vi "FTW-TestExecutive-Core_OnLoadSequence.vi"(0 "FTW-Scripter-Core In":refnum<class "FTW-TestExecutive-Core.lvclass">, 11 "error in":errorcluster) -> (4 "FTW-Scripter-Core Out":refnum<class "FTW-TestExecutive-Core.lvclass">, 15 "error out":errorcluster)   [LabVIEW 2015, in "FTW-TestExecutive-Core.lvclass"]
uses:
  FTW-TestExecutive-Core.lvclass
  FTW-TestExecutive-Core.lvclass/FTW-TestExecutive-Core.ctl
  source/actor/Instance-Extended/FTW-ActorExtended.lvclass
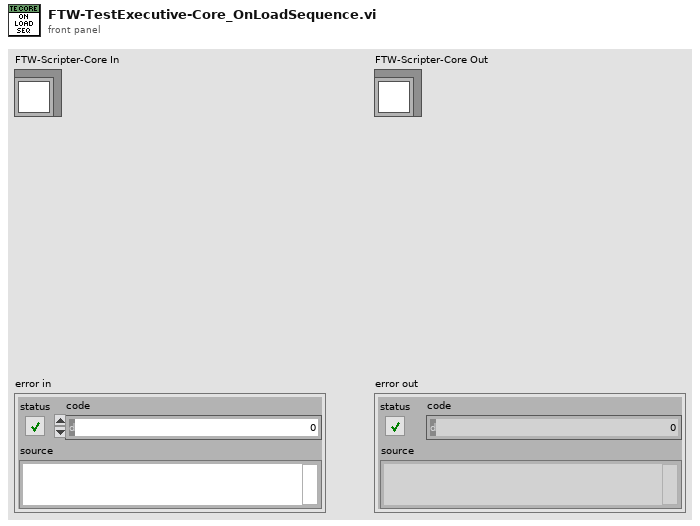
[diagram p1: front panel]
types:
  T1 = typedef "FTW-TestExecutive-Step.ctl" = cluster{"Name":string, "Type":string, "Path":string, "Config":string, "Elapsed Time":dbl, "Passed":bool, "State":T2, "Results":T3}
  T2 = typedef "FTW-TestExecutive-Step-State.ctl" = enum8{"None", "Failed", "Passed", "Timed out", "Aborted"}
  T3 = typedef "FTW-TestExecutive-Results.ctl" = cluster{"Start Time":timestamp, "Elapsed Time":dbl, "Passed":bool, "Additional Results":refnum<class "FTW-Container.lvclass">}
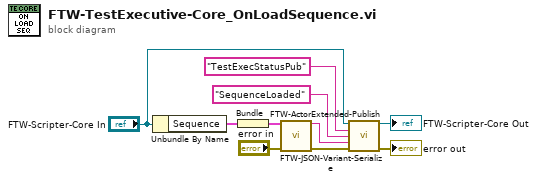
[diagram p0: block diagram]
diagram:
  n1 = Unbundle By Name("FTW-Scripter-Core In") -> ("Sequence"=w1:T1[])
  n2 = Bundle("Sequence"=w1) -> (w2:cluster{"Sequence":T1[]})  [unwired: 1 in]
  n3 = call "FTW-JSON-Variant-Serialize.vi"("Variant"=w2, "error in"="error in") -> ("JSON String"=w3:string, "error out"=w4:errorcluster)  [unwired: 12 in]
  n4 = call "FTW-ActorExtended-Publish.vi"("FTW-ActorExtended In"="FTW-Scripter-Core In", "Publisher Name"="TestExecStatusPub", "Message Header"="SequenceLoaded", "Message Body"=w3, "error in"=w4) -> ("FTW-ActorExtended Out"=→"FTW-Scripter-Core Out":refnum<class "FTW-TestExecutive-Core.lvclass">, "error out"=→"error out":errorcluster)  [unwired: 9 in]
